vi "Shutter control.vi"(4 "error in (no error)":errorcluster, 5 "input main cluster":T1, 7 "shutter control":bool) -> (0 "error out":errorcluster, 1 "input main cluster":T1)   [LabVIEW 2010]
uses:
  <vilib>/DAQmx/write.llb/DAQmx Write (Digital Bool 1Line 1Point).vi
  Main_cluster.ctl
  <vilib>/vision/Image Controls.llb/IMAQ Image.ctl
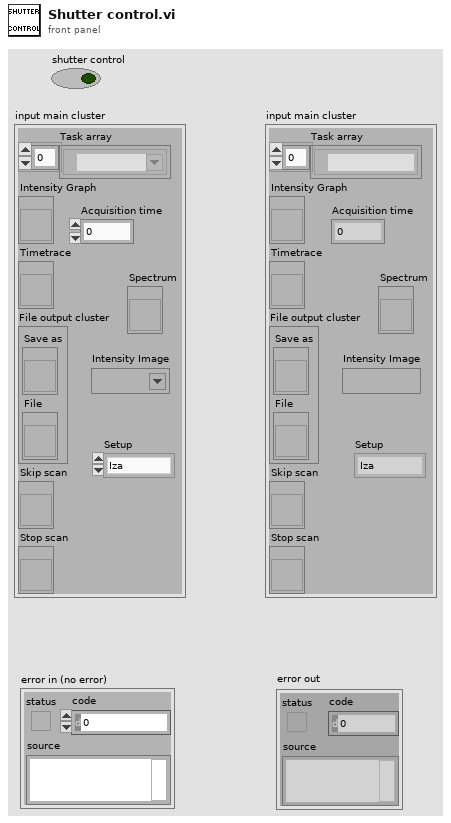
[diagram p1: front panel]
types:
  T1 = typedef "Main_cluster.ctl" = cluster{"Task array":refnum<k21>[], "Intensity Graph":refnum<vi>, "Timetrace":refnum<vi>, "File output cluster":cluster{"Save as":refnum<vi>, "File":refnum<vi>}, "Skip scan":refnum<vi>, "Stop scan":refnum<vi>, "Acquisition time":dbl, "Setup":enum16{"Iza", "Lukasz"}, "Spectrum":refnum<vi>, "Intensity Image":T2}
  T2 = typedef "IMAQ Image.ctl" = refnum<image>
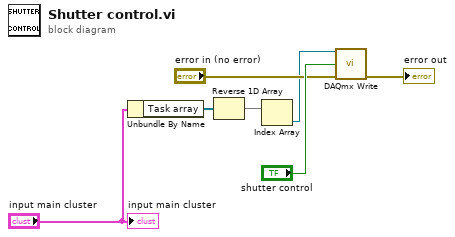
[diagram p0: block diagram]
diagram:
  n1 = Unbundle By Name("input main cluster") -> ("Task array"=w4:refnum<k21>[])
  n2 = Reverse 1D Array(array=w4) -> (reversed array=w1:refnum<k21>[])
  n3 = Index Array(array=w1) -> (element=w5:refnum<k21>)  [unwired: 1 in]
  n4 = call-poly <vilib>:"DAQmx Write.vi"("task/channels in"=w5, "data"="shutter control", "error in"="error in (no error)") -> ("error out"=→"error out":errorcluster)  [unwired: 10 in, 2 out]
  "input main cluster" <- "input main cluster"
